vi "8CHDAQ - Scale Data.vi"(10 "Array Input":dbl[][](array[numeric]), 11 "Channel Data":T1) -> (3 "Array Output":dbl[][](array[numeric]))   [LabVIEW 2015]
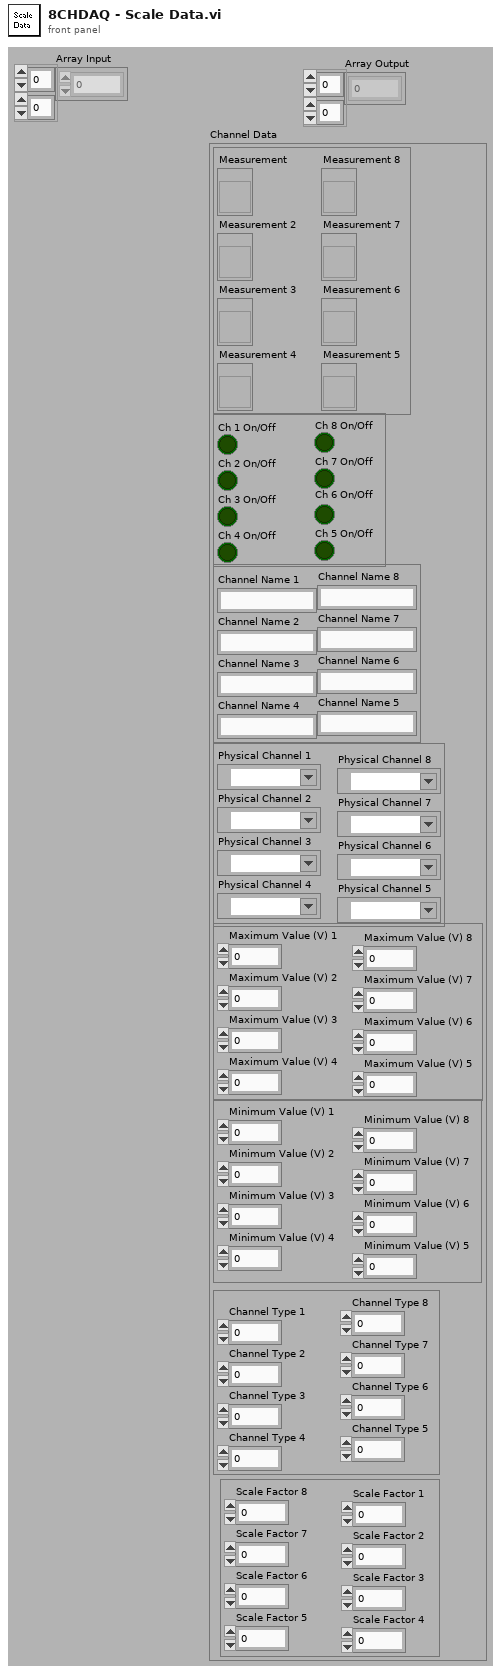
[diagram p1: front panel]
types:
  T1 = cluster{cluster{"Measurement":refnum<vi>, "Measurement 2":refnum<vi>, "Measurement 3":refnum<vi>, "Measurement 4":refnum<vi>, "Measurement 5":refnum<vi>, "Measurement 6":refnum<vi>, "Measurement 7":refnum<vi>, "Measurement 8":refnum<vi>}, cluster{"Ch 1 On/Off":bool, "Ch 2 On/Off":bool, "Ch 3 On/Off":bool, "Ch 4 On/Off":bool, "Ch 5 On/Off":bool, "Ch 6 On/Off":bool, "Ch 7 On/Off":bool, "Ch 8 On/Off":bool}, cluster{"Channel Name 1":string, "Channel Name 2":string, "Channel Name 3":string, "Channel Name 4":string, "Channel Name 5":string, "Channel Name 6":string, "Channel Name 7":string, "Channel Name 8":string}, cluster{"Physical Channel 1":tag, "Physical Channel 2":tag, "Physical Channel 3":tag, "Physical Channel 4":tag, "Physical Channel 5":tag, "Physical Channel 6":tag, "Physical Channel 7":tag, "Physical Channel 8":tag}, cluster{"Maximum Value (V) 1":dbl, "Maximum Value (V) 2":dbl, "Maximum Value (V) 3":dbl, "Maximum Value (V) 4":dbl, "Maximum Value (V) 5":dbl, "Maximum Value (V) 6":dbl, "Maximum Value (V) 7":dbl, "Maximum Value (V) 8":dbl}, cluster{"Minimum Value (V) 1":dbl, "Minimum Value (V) 2":dbl, "Minimum Value (V) 3":dbl, "Minimum Value (V) 4":dbl, "Minimum Value (V) 5":dbl, "Minimum Value (V) 6":dbl, "Minimum Value (V) 7":dbl, "Minimum Value (V) 8":dbl}, cluster{"Channel Type 1":u16, "Channel Type 2":u16, "Channel Type 3":u16, "Channel Type 4":u16, "Channel Type 5":u16, "Channel Type 6":u16, "Channel Type 7":u16, "Channel Type 8":u16}, cluster{"Scale Factor 8":dbl[unit], "Scale Factor 7":dbl[unit], "Scale Factor 6":dbl[unit], "Scale Factor 5":dbl[unit], "Scale Factor 4":dbl[unit], "Scale Factor 3":dbl[unit], "Scale Factor 2":dbl[unit], "Scale Factor 1":dbl[unit]}}
  T2 = cluster{"Channel Type 1":u16, "Channel Type 2":u16, "Channel Type 3":u16, "Channel Type 4":u16, "Channel Type 5":u16, "Channel Type 6":u16, "Channel Type 7":u16, "Channel Type 8":u16}
  T3 = cluster{"Scale Factor 8":dbl[unit], "Scale Factor 7":dbl[unit], "Scale Factor 6":dbl[unit], "Scale Factor 5":dbl[unit], "Scale Factor 4":dbl[unit], "Scale Factor 3":dbl[unit], "Scale Factor 2":dbl[unit], "Scale Factor 1":dbl[unit]}
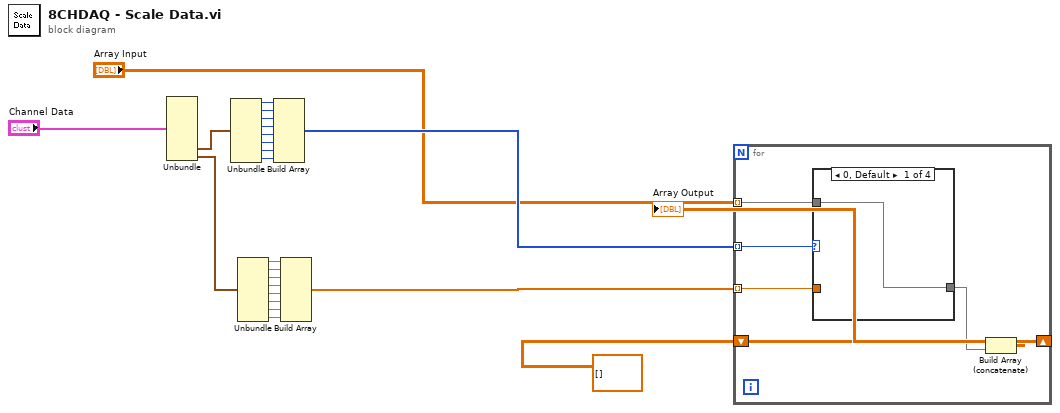
[diagram p0: block diagram]
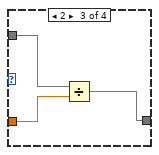
[diagram p3: hidden frame]
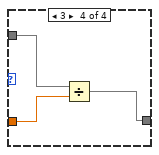
[diagram p4: hidden frame]
diagram:
  n1 = Unbundle("Channel Data") -> (w24:T2, w13:T3)  [unwired: 6 out]
  n2 = Unbundle(w24) -> ("Channel Type 1"=w23:u16, "Channel Type 2"=w22:u16, "Channel Type 3"=w21:u16, "Channel Type 4"=w20:u16, "Channel Type 5"=w5:u16, "Channel Type 6"=w6:u16, "Channel Type 7"=w7:u16, "Channel Type 8"=w8:u16)
  n3 = Unbundle(w13) -> ("Scale Factor 8"=w17:dbl[unit], "Scale Factor 7"=w16:dbl[unit], "Scale Factor 6"=w15:dbl[unit], "Scale Factor 5"=w14:dbl[unit], "Scale Factor 4"=w1:dbl[unit], "Scale Factor 3"=w2:dbl[unit], "Scale Factor 2"=w3:dbl[unit], "Scale Factor 1"=w4:dbl[unit])
  n4 = Build Array(w23, w22, w21, w20, w5, w6, w7, w8) -> (w19:u16[])
  n5 = Build Array(w17, w16, w15, w14, w1, w2, w3, w4) -> (w12:dbl[])
  n6 = for {
    tunnel: w19 -> [w30] mode=indexing
    shift-right: [w28] -> w11
    shift-left: dbl[][] [] -> [w29]
    tunnel: w12 -> [w27] mode=indexing
    tunnel: "Array Input" -> [w26] mode=indexing
    n7 = case shown="0, Default" w30 {
      tunnel: [w31 w32 w35 w38] -> w25
      tunnel: w27 -> [_ _ w33 w36]
      tunnel: w26 -> [w31 w32 w34 w37]
      frame 0, Default {
      }
      frame 1 {
      }
      frame 2 {
        n8 = Divide(x=w34, y=w33) -> (x/y=w35:dbl[])
      }
      frame 3 {
        n9 = Divide(x=w37, y=w36) -> (x/y=w38:dbl[])
      }
    }
    n10 = Build Array (concatenate)(w29, w25) -> (w28:dbl[][])
  }
  "Array Output" <- w11
